vi "SetDC Offset.vi"(6 "DC offset [V]":dbl caption="DC offset", 8 "error in (no error)":errorcluster, 9 "channel":i32, 10 "Fpga input":T1, 11 "Scope5785_six_channel":refnum<class "Scope5782_six_channel.lvclass">) -> (0 "error out":errorcluster, 3 "Scope5785_six_channel out":refnum<class "Scope5782_six_channel.lvclass">)   [LabVIEW 2025, in "Scope5782_six_channel.lvclass"]
uses:
  Scope5782_six_channel.lvclass
  fpga ID.ctl
  Scope5782_six_channel.lvclass/Scope5782_six_channel.ctl
  FPGA/fpga_settings.ctl
  FpgaRef/FpgaRef5761/FpgaRef5761.lvclass
  FpgaRef/FpgaRefx410/FpgaRefx410.lvclass
  <vilib>/rvi/FXPMathLib/FxpInterpret/XNode/nifxpmath_Interpret.xnode
  C:/PXIe/InProgress/source/Host/FpgaRef/FpgaRefBase/FpgaRefBase.lvclass
  C:/PXIe/InProgress/source/Host/FpgaRef/FpgaRef5761/FpgaRef5761.lvclass
  C:/PXIe/InProgress/source/Host/FpgaRef/FpgaRefx410/FpgaRefx410.lvclass
  FpgaRef/FpgaRefBase/FpgaRefBase.lvclass
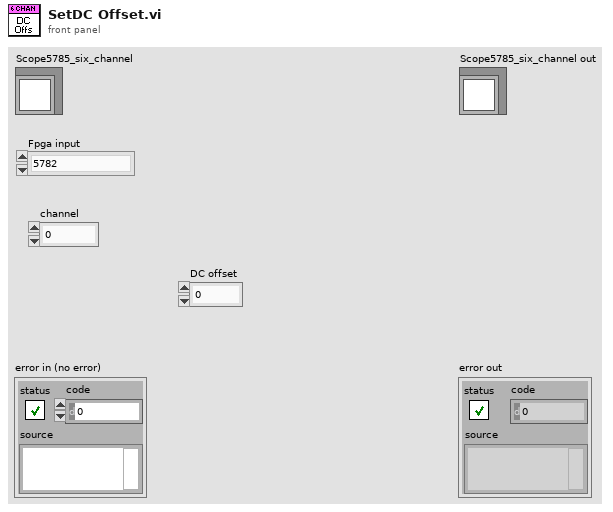
[diagram p1: front panel]
types:
  T1 = typedef "Scope5782_six_channel.lvclass/fpga ID.ctl" = enum16{"5782", "5761"}
  T2 = typedef "fpga_settings.ctl" = enum16{"Feedback Enable", "New FIR coeffs", "FIR shift", "Enable filter", "Set Downsample", "Downsample", "CIC Gain", "Record length", "Trigger samples", "Quiet time", "a_am", "b_am", "Use fixed delay", "fixed sin_fi", "fixed cos_fi", "Ki*Tau", "Kp", "Kd_Tau", "Fi_start", "Fi_delta", "DC_offs 0", "DC_offs 1", "DC_offs 2", "DC_offs 3", "Ki*Tau am", "Kp am", "Kd_Tau am", "Feedback AM", "Trigger delay", "Feedback delay", "Setpoint enable", "Beam enable", "Samples to acquire", "Cavity Enable", "Cavity C1", "Cavity C2", "Cavity C3", "Cavity C4", "Cavity C5", "Input delay", "Ki*Tau Q", "Kp Q", "Kd_Tau Q", "Adaptive FF enable", "Feedforward a0", "Feedforward b0", "FF src adress", "FF dest adress", "Output scale", "Input scale", "Host scale", "FF_IIR b0", "FF_IIR b1", "FF_IIR b2", "FF_IIR-a1", "FF_IIR-a2", "Enable HW trigger", "Virtual cavity", "Samples to skip", "Samples to skip 2", "Samples to skip 3", "Cavity C3_2", "Cavity C4_2", "Cavity C5_2", "Cavity C3_3", "Cavity C4_3", "Cavity C5_3", "Cavity_w0_dt", "Piezo setting", "Quench t0", "Quench tau set", "Quench enabled", "Quench reset", "PID enabled I", "PID enabled Q", "Cavity filter a", "Cavity filter b", "Disable e(n)", "FF e(n) src address", "FF first address", "FF last address", "FF PID first address", "FF PID last address", "Amp IIR b0", "Amp IIR b1", "Amp IIR b2", "Amp IIR-a1", "Amp IIR-a2", "Adaptation factor", "Inv Amp LP b0", "Inv Amp LP b1", "Inv Amp LP b2", "Inv Amp LP-a1", "Inv Amp LP-a2", "Inv Amp c0", "Inv Amp c1", "Inv Amp c2", "Inv Amp c3", "Inv Amp c4", "Inv Amp -d1", "Inv Amp -d2", "Inv Amp -d3", "Inv Amp -d4", "w12_a", "w12_b", "w12_dt", "w12_scale", "dw_scale", "Extra output select", "Extra fi sin", "Extra fi cos", "Extra output scale", "Quench max output"}
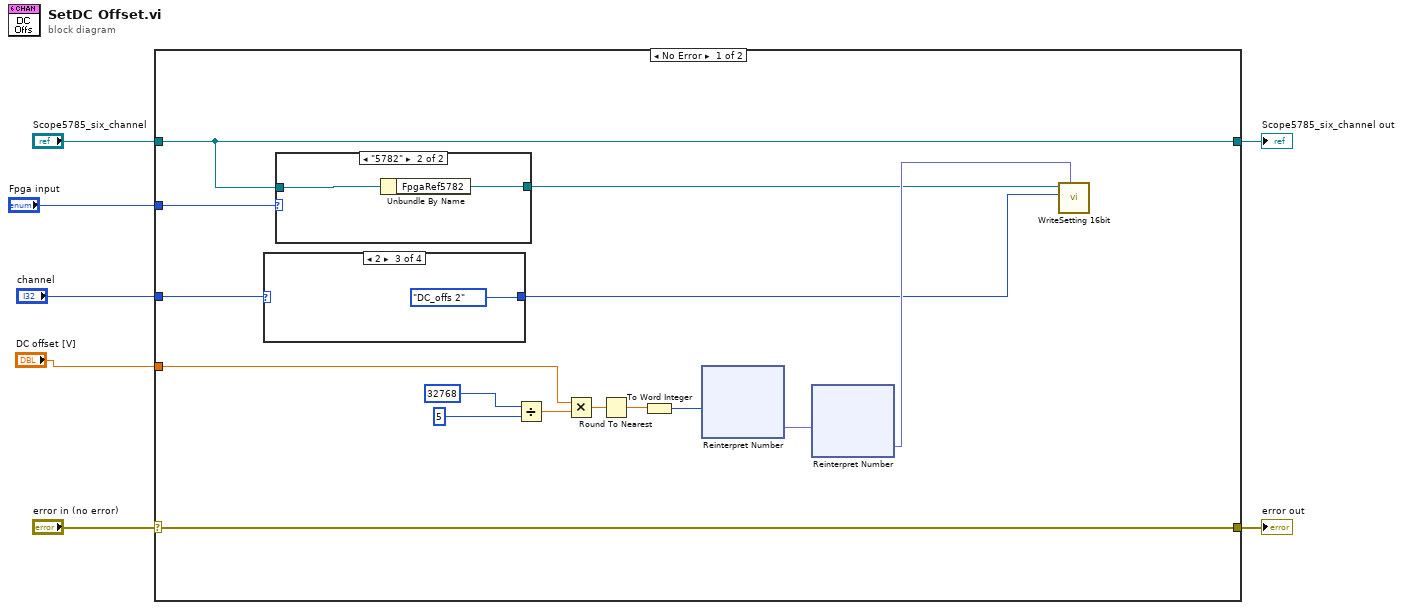
[diagram p0: block diagram]
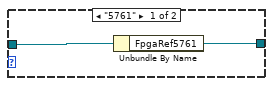
[diagram p2: hidden frame]
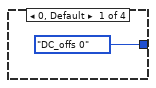
[diagram p3: hidden frame]
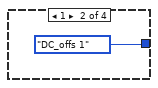
[diagram p4: hidden frame]
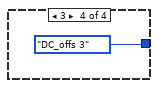
[diagram p5: hidden frame]
diagram:
  n1 = case shown="No Error" "error in (no error)" {
    selector: "error in (no error)" -> [w22 w32]
    tunnel: [w22 w32] -> w6
    tunnel: [w10 w31] -> w4
    tunnel: "Scope5785_six_channel" -> [w10 w31]
    tunnel: "DC offset [V]" -> [w14 _]
    tunnel: "channel" -> [w13 _]
    tunnel: "Fpga input" -> [w11 _]
    frame No Error {
      n2 = case shown="2" w13 {
        tunnel: [fpga_settings."DC_offs 0" ("FPGA Setting") fpga_settings."DC_offs 1" ("FPGA Setting") fpga_settings."DC_offs 2" ("FPGA Setting") fpga_settings."DC_offs 3" ("FPGA Setting")] -> w8
        frame 0, Default {
        }
        frame 1 {
        }
        frame 2 {
        }
        frame 3 {
        }
      }
      n3 = case shown="\"5782\"" w11 {
        tunnel: w10 -> [w24 w26]
        tunnel: [w23 w25] -> w9
        frame "5761" {
          n4 = Unbundle By Name(w24) -> ("FpgaRef5761"=w23:refnum<class "FpgaRef5761.lvclass">)
        }
        frame "5782" {
          n5 = Unbundle By Name(w26) -> ("FpgaRef5782"=w25:refnum<class "FpgaRefx410.lvclass">)
        }
      }
      n6 = Divide(x=32768, y=5) -> (x/y=w19:dbl)
      n7 = Multiply(x=w14, y=w19) -> (x*y=w18:dbl)
      n8 = Round To Nearest(number=w18) -> (nearest integer value=w17:dbl)
      n9 = To Word Integer(number=w17) -> (16bit integer=w16:i16)
      n10 = xnode "Reinterpret Number"("x"=w16) -> ("y"=w15:fxp<+/-,16,14>)
      n11 = xnode "Reinterpret Number"("x"=w15) -> ("y"=w12:fxp<+,16,16>)
      n12 = call "WriteSetting 16bit.vi"("value"=w12, "FPGA Setting"=w8, "FpgaRefBase in"=w9) -> ()  [unwired: 7 in, 2 out]
    }
    frame Error {
    }
  }
  "error out" <- w6
  "Scope5785_six_channel out" <- w4
